vi "Main.vi"(9 "Robot Initial Position\nFrom Simulator SW corner":T1={"East"=20.0, "North"=20.0}, 10 "Simulator Bounds":T2={"Simulator E Range"=20.0, "Simulator E Min"=-10.0, "Simulator N Range"=20.0, "Simulator N Min"=-10.0}, 11 "Which Boat Am I?\n(unnecessary to set on RIO)":T3=enum."Simulation") -> ()   [LabVIEW 2011]
doc: "The main VI for Sense, Think and Act that controls the sailbot. Also includes logging code and code for communication with the OCU.\nby Olin Sailbot\noriginally by Jason Curtis"
uses:
  2-Think/2 Typedefs/Which Boat.ctl
  1,3 B-Simulation/1,3 B Typedefs/simulator bounds.ctl
  2-Think/2 Typedefs/robot velocity.ctl
  2-Think/2 Typedefs/setpoints to boat.ctl
  2-Think/2 Typedefs/sail setpt.ctl
  2-Think/2 Typedefs/rudder angle.ctl
  2-Think/2 Typedefs/UTM Circle.ctl
  0x2-OCU-Think Comm/0x2 Typedefs/Waypoints List.ctl
  2-Think/2 Classes/Waypoint/Waypoint.lvclass
  0x2-OCU-Think Comm/0x2 Typedefs/Current Waypoint.ctl
  2-Think/2 Typedefs/eStopCommand.ctl
  0x2-OCU-Think Comm/0x2 Typedefs/ocuMessage.ctl
  0x2-OCU-Think Comm/0x2 Typedefs/ocuCommands.ctl
  <vilib>/Platform/TimedLoop/XDataNode/timing_clust.ctl
  <vilib>/Platform/TimedLoop/XDataNode/nitl_modes.ctl
  <vilib>/Platform/TimedLoop/XDataNode/wakeup.ctl
  2-Think/2 Globals/2 Global.vi
  2-Think/2 Globals/2 Message Logger.vi
  <vilib>/Platform/TimedLoop/XDataNode/XDataNode.xnode
  <vilib>/Platform/TimedLoop/XDataNode/XDNodeRunTimeDep.lvlib
  0x2-OCU-Think Comm/0x2 Classes/NetworkStreams/Writer/NetworkStreamWriter.lvclass
  0x2-OCU-Think Comm/0x2 Classes/NetworkStreams/Reader/NetworkStreamReader.lvclass
  2-Think/2 Classes/Logger/Logger.lvclass
panel:
  in  "Skip Sense (->manual input only!)":bool
  in  "Enable logging?":bool=TRUE
  in  "Data storage folder":path
  out "E-stop freq.":dbl
  out "Act freq.":dbl
  out "Sense freq.":dbl
  out "Think freq.":dbl
  in  "E-Stop":bool
  # "this is the parent VI under which \nSense Think and Act run."
  # "Will save to U:\\Logs when run on the RIO"
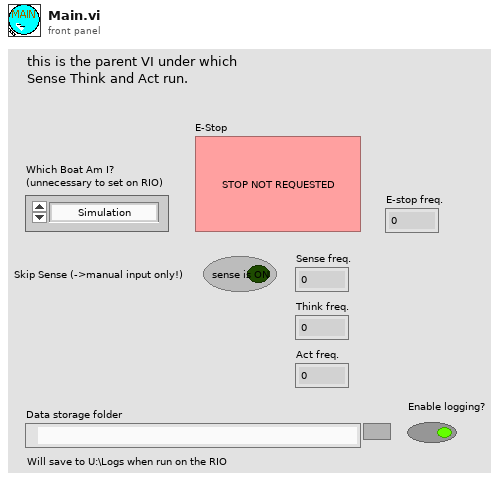
[diagram p1: front panel]
types:
  T1 = typedef "robot velocity.ctl" = cluster{"East":dbl, "North":dbl}
  T2 = typedef "simulator bounds.ctl" = cluster{"Simulator E Range":dbl, "Simulator E Min":dbl, "Simulator N Range":dbl, "Simulator N Min":dbl}
  T3 = typedef "Which Boat.ctl" = enum16{"Competition Boat", "Small RC", "Simulation"}
  T4 = typedef "setpoints to boat.ctl" = cluster{"Sail Position":T5, "Rudder Angle":T6}
  T5 = typedef "sail setpt.ctl" = dbl
  T6 = typedef "rudder angle.ctl" = dbl
  T7 = typedef "UTM Circle.ctl" = cluster{"UTM Zone":dbl, "Hemisphere":enum16{"North", "South"}, "East":dbl, "North":dbl, "Radius":dbl}
  T8 = typedef "Waypoints List.ctl" = refnum<class "Waypoint.lvclass">[]
  T9 = typedef "Current Waypoint.ctl" = i32
  T10 = typedef "eStopCommand.ctl" = enum16{"Reset E-Stop", "Get E-Stop", "Set E-Stop"}
  T11 = typedef "ocuMessage.ctl" = cluster{"OCU Command":T12, "Data":variant}
  T12 = typedef "ocuCommands.ctl" = enum16{"Pass", "Send override", "Add waypoint", "Set waypoint number", "Stop", "Add Mission", "Reset Missions/Waypts", "Edit Control Values", "Add Global No-Sail", "Log Message"}
  T13 = typedef "XDNodeRunTimeDep.lvlib/timing_clust.ctl" = cluster{"Expected End [f-1]":u64, "Actual End [f-1]":u64, "Finished Late? [f-1]":bool, "Expected End [i-1]":u64, "Actual End [i-1]":u64, "Finished Late? [i-1]":bool, "Expected Start [i]":u64, "Actual Start [i]":u64, "Expected Start [f]":u64, "Actual Start [f]":u64, "Source Name":string, "Structure Name":string, "Period":i64, "Deadline":i64, "Offset":i64, "Start":i64, "Priority":i32, "Timeout":i32, "Mode":T14, "Wakeup Reason":T15, "Error":errorcluster, "Source Type":string, "Secondary Source Type":string, "Global End Time":u64, "Global Start Time":u64, "Frame Duration":u64, "Iteration Duration":u64, "Assigned CPU":i32, "I/O Scan Engine Mode":u32}
  T14 = typedef "XDNodeRunTimeDep.lvlib/nitl_modes.ctl" = enum32{"No Change", "Process missed periods, maintain original phase", "Discard missed periods, maintain original phase", "Process missed periods, ignore original phase", "Discard missed periods, ignore original phase"}
  T15 = typedef "XDNodeRunTimeDep.lvlib/wakeup.ctl" = enum32{"Normal", "Aborted", "Asynchronous wakeup", "Timing source error", "Timed loop error", "Timeout"}
  T16 = typedef "IMAQ Image.ctl" = refnum<image>
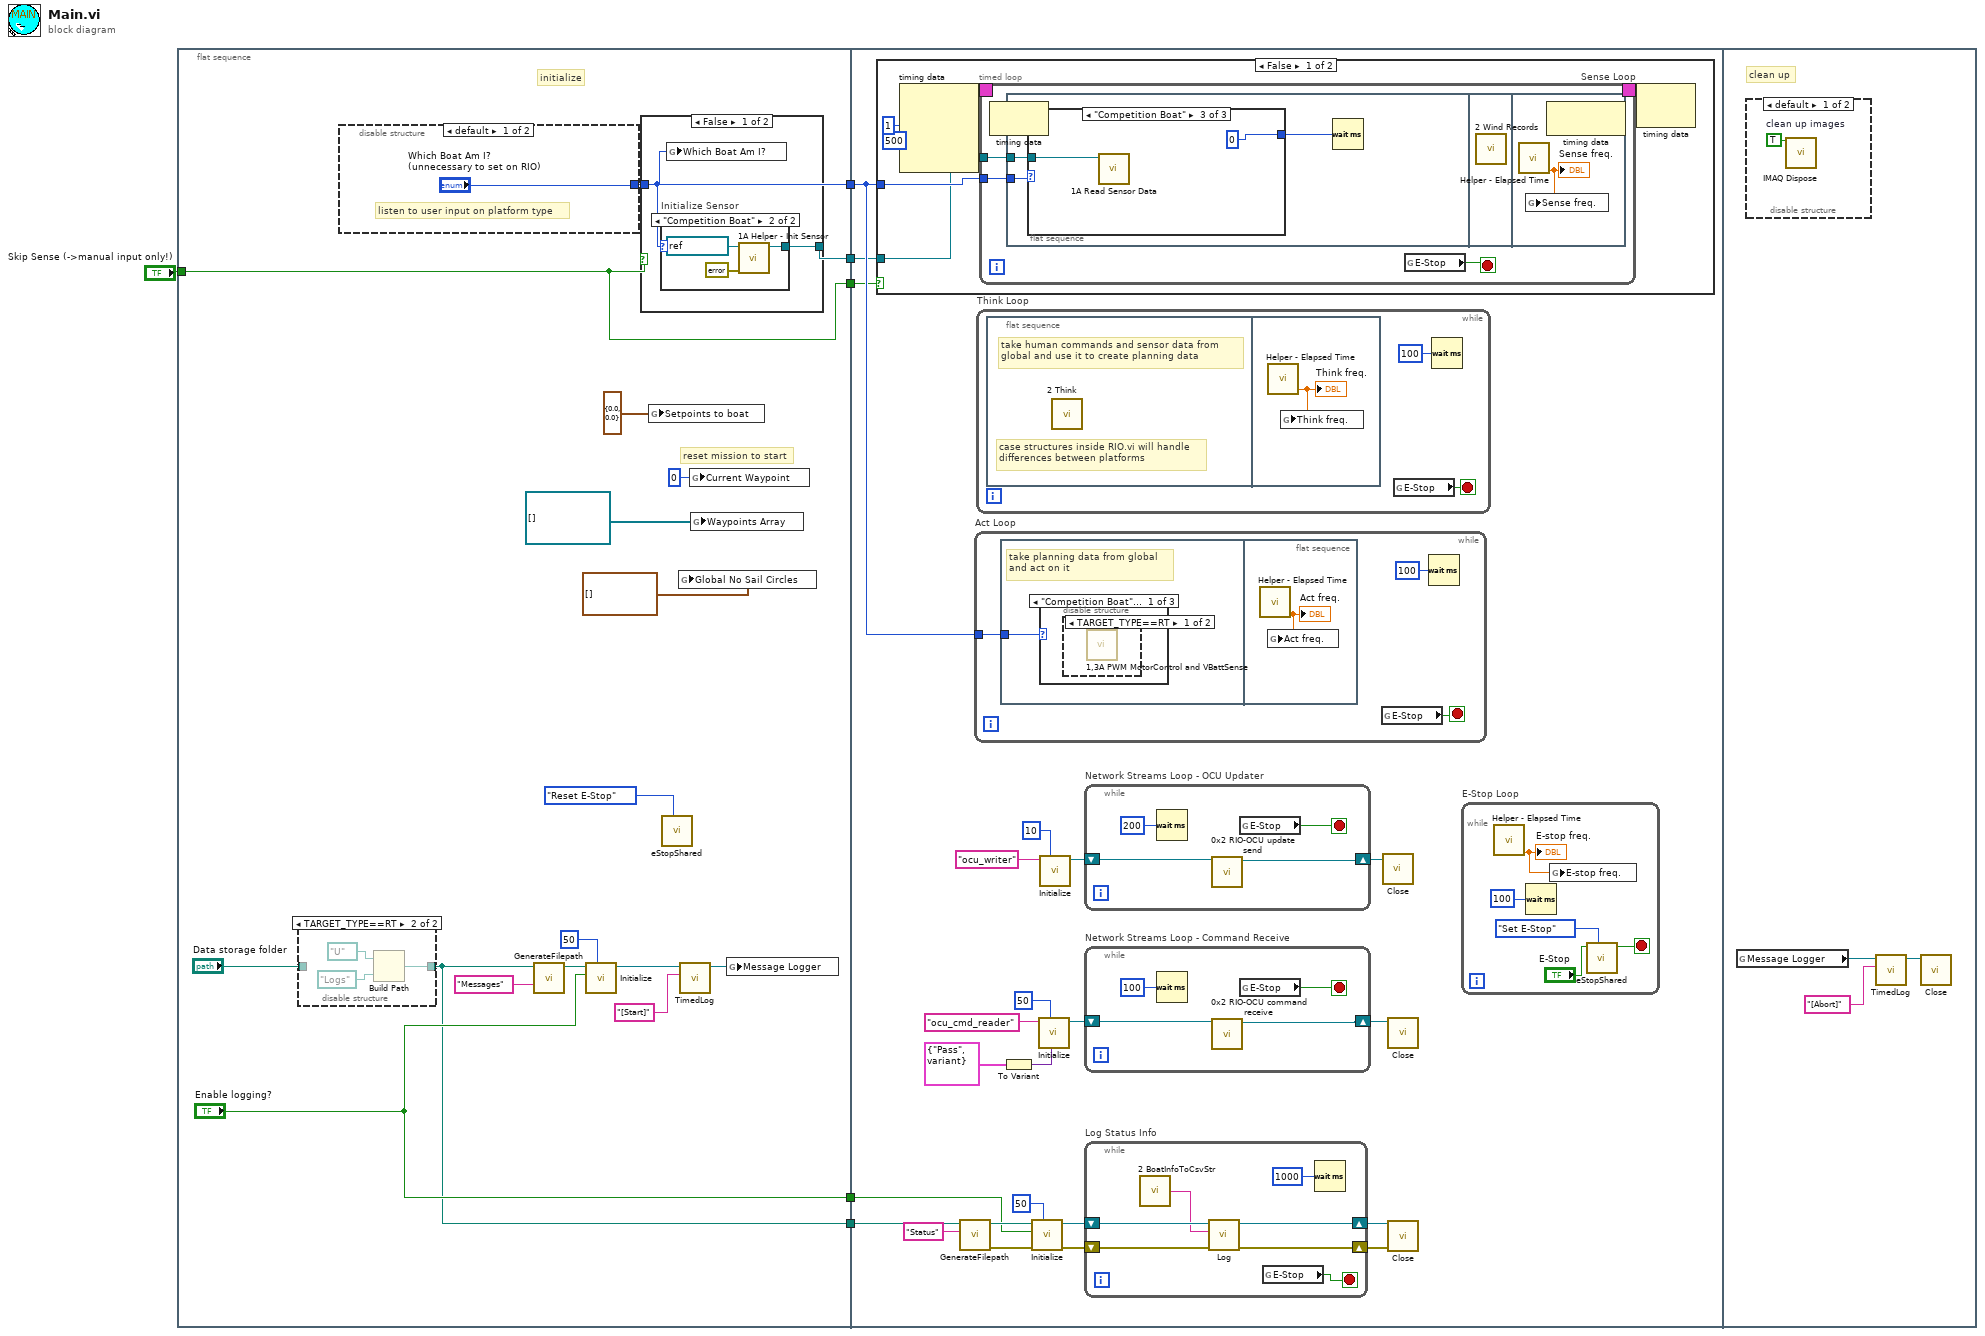
[diagram p0: block diagram]
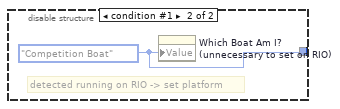
[diagram p5: hidden frame]
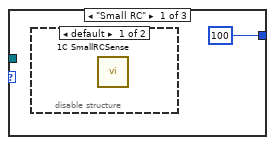
[diagram p6: hidden frame]
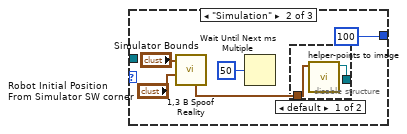
[diagram p8: hidden frame]
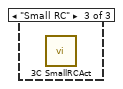
[diagram p13: hidden frame]
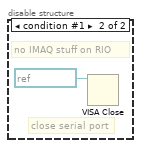
[diagram p14: hidden frame]
diagram:
  n1 = flat-sequence {
    tunnel: [w20] -> w6
    tunnel: [w21] -> w5
    tunnel: [w14] -> w4
    tunnel: ["Enable logging?"] -> w3
    tunnel: "Skip Sense (->manual input only!)" -> [w12]
    tunnel: [w12] -> w1
    tunnel: w6 -> [w57]
    tunnel: w5 -> [w56]
    tunnel: w4 -> [w40]
    tunnel: w3 -> [w36]
    tunnel: w1 -> [w35]
    frame #0 {
      # "reset mission to start"
      # "initialize"
      n2 = disable-structure shown="TARGET_TYPE==RT" {
        disable-tunnel: "Data storage folder" -> [w29 _]
        disable-tunnel: [w29 w30] -> w14
        frame condition #0 (active) {
        }
        frame condition #1 {
          n3 = Build Path(base path=path "U:/" ("Data storage folder"), name or relative path=path "Logs" ("Data storage folder")) -> (appended path=w30:path)
        }
      }
      n4 = disable-structure shown="default" {
        disable-tunnel: ["Which Boat Am I?\n(unnecessary to set on RIO)" w34] -> w20
        frame condition #0 (active) {
          # "listen to user input on platform type"
        }
        frame condition #1 {
          w34 = Which_Boat."Competition Boat" ("Which Boat Am I?")
          # "detected running on RIO -> set platform"
          n5 = property on="Which Boat Am I?\n(unnecessary to set on RIO)" class="Enum (strict)"("Value"=w34) -> ()  [unwired: 2 in, 2 out]
        }
      }
      n6 = call "GenerateFilepath.vi"("Identifier"="Messages", "Data storage folder"=w14) -> ("File path out"=w17:path)  [unwired: 8 in, 1 out]
      n7 = call "Initialize.vi"("buffer size"=50, "Enable? (T)"="Enable logging?", "File path"=w17) -> ("Logger out"=w9:refnum<class "Logger.lvclass">)  [unwired: 7 in, 1 out]
      n8 = case shown="False" w12 {
        tunnel: [w25 _] -> w21
        tunnel: w20 -> [w24 _]
        frame False {
          n9 = case "Initialize Sensor" shown="\"Competition Boat\"" w24 {
            tunnel: [_ w26] -> w25
            frame Default {
            }
            frame "Competition Boat" {
              n10 = call "1A Helper - Init Sensor.vi"("error in (no error)"=errorcluster {"status"=FALSE, "code"=0, "source"=""}, "VISA Refnum in"=refnum<visa-resource-name> "COM1" ("VISA resource name")) -> ("VISA Refnum out"=w26:refnum<visa-resource-name>)  [unwired: 7 in, 2 out]
            }
          }
          n11 = global write "2 Global.vi" "Which Boat Am I?"(w24) -> ()
        }
        frame True {
        }
      }
      n12 = global write "2 Global.vi" "Setpoints to boat"(T4 {"Sail Position"=0.0, "Rudder Angle"=0.0} ("Setpoints to boat")) -> ()
      n13 = call "eStopShared.vi"("Command"=eStopCommand."Reset E-Stop") -> ()  [unwired: 9 in, 2 out]
      n14 = global write "2 Global.vi" "Global No Sail Circles"(T7[] [] ("Global No Sail Circles")) -> ()
      n15 = call "TimedLog.vi"("Message"="[Start]", "Logger in"=w9) -> ("Logger out"=w8:refnum<class "Logger.lvclass">)  [unwired: 7 in, 2 out]
      n16 = global write "2 Global.vi" "Current Waypoint"(T9 0 ("Current Waypoint")) -> ()
      n17 = global write "2 Global.vi" "Waypoints Array"(T8 [] ("Waypoints Array")) -> ()
      n18 = global write "2 Message Logger.vi" "Message Logger"(w8) -> ()
    }
    frame #1 {
      n19 = case shown="False" w35 {
        tunnel: w57 -> [w61 _]
        tunnel: w56 -> [w60 _]
        frame False {
          n20 = node-c288(i64 1 ("Period"), 500 ("Priority")) -> (w63:T13)  [unwired: 2 in]
          n21 = timed-loop "Sense Loop" {
            tunnel: w61 -> [w65]
            tunnel: w60 -> [w64]
            timing: w63 -> [_]
            timing-out: [_] -> w62
            stop <- w66 stop-if-true
            n22 = node-c288() -> ()  [unwired: 1 in, 1 out]
            n23 = flat-sequence {
              tunnel: w65 -> [w71]
              tunnel: w64 -> [w69]
              frame #0 {
                n24 = case shown="\"Competition Boat\"" w71 {
                  tunnel: [u32 100 ("millisecond multiple") u32 100 ("millisecond multiple") u32 0 ("millisecond multiple")] -> w70
                  tunnel: w69 -> [_ _ w80]
                  frame "Small RC" {
                    n25 = disable-structure shown="default" {
                      frame condition #0 (active) {
                        n26 = call "1C SmallRCSense.vi"() -> ()  [unwired: 6 in, 6 out]
                      }
                      frame condition #1 {
                      }
                    }
                  }
                  frame "Simulation" {
                    n27 = call "1,3 B Spoof Reality.vi"("Robot Initial Position\nFrom Simulator SW corner"="Robot Initial Position\nFrom Simulator SW corner", "Simulator Bounds"="Simulator Bounds") -> ("Boat Path"=w76:cluster{"X Position":dbl, "Y Position":dbl}[])  [unwired: 3 in, 6 out]
                    n28 = Wait Until Next ms Multiple(millisecond multiple=u32 50) -> ()  [unwired: 1 out]
                    n29 = disable-structure shown="default" {
                      disable-tunnel: w76 -> [w79 _]
                      disable-tunnel: [w78 _] -> _
                      frame condition #0 (active) {
                        n30 = call "helper-points to image.vi"("Array of Points"=w79) -> ("Image Out"=w78:T16)  [unwired: 10 in]
                      }
                      frame condition #1 {
                        # "no IMAQ\non RIO"
                      }
                    }
                  }
                  frame "Competition Boat" {
                    n31 = call "1A Read Sensor Data.vi"("VISA resource name (in)"=w80) -> ()  [unwired: 9 in, 2 out]
                  }
                }
                n32 = Wait (ms)(milliseconds to wait=w70) -> ()  [unwired: 1 out]
              }
              frame #1 {
                n33 = call "2 Wind Records.vi"() -> ()  [unwired: 12 in]
              }
              frame #2 {
                n34 = call "Helper - Elapsed Time.vi"() -> ("Frequency (Hz)"=w82:dbl)  [unwired: 10 in, 1 out]
                "Sense freq." <- w82
                n35 = global write "2 Global.vi" "Sense freq."(w82) -> ()
              }
            }
            n36 = global read "2 Global.vi" "E-Stop"() -> (w66:bool)
            n37 = node-c288() -> ()  [unwired: 1 in, 1 out]
          }
          n38 = node-c288(w62) -> ()  [unwired: 1 out]
        }
        frame True {
          # "Sense is cancelled"
        }
      }
      n39 = call "GenerateFilepath.vi"("Identifier"="Status", "Data storage folder"=w40) -> ("error out"=w44:errorcluster, "File path out"=w45:path)  [unwired: 8 in]
      n40 = while "Act Loop" {
        tunnel: w57 -> [w112]
        stop <- w113 stop-if-true
        n41 = flat-sequence {
          tunnel: w112 -> [w114]
          frame #0 {
            # "take planning data from global\nand act on it"
            n42 = case shown="\"Competition Boat\", Default" w114 {
              frame "Competition Boat", Default {
                n43 = disable-structure shown="TARGET_TYPE==RT" {
                  frame condition #0 {
                    n44 = call "1,3A PWM MotorControl and VBattSense.vi"() -> ()  [unwired: 12 in]
                  }
                  frame condition #1 (active) {
                  }
                }
              }
              frame "Simulation" {
                # "simulation Act\nis integrated with\nsimulation Think"
              }
              frame "Small RC" {
                n45 = call "3C SmallRCAct.vi"() -> ()  [unwired: 12 in]
              }
            }
          }
          frame #1 {
            n46 = call "Helper - Elapsed Time.vi"() -> ("Frequency (Hz)"=w115:dbl)  [unwired: 10 in, 1 out]
            "Act freq." <- w115
            n47 = global write "2 Global.vi" "Act freq."(w115) -> ()
          }
        }
        n48 = global read "2 Global.vi" "E-Stop"() -> (w113:bool)
        n49 = Wait (ms)(milliseconds to wait=u32 100 ("millisecond multiple")) -> ()  [unwired: 1 out]
      }
      n50 = while "Think Loop" {
        stop <- w109 stop-if-true
        n51 = flat-sequence {
          frame #0 {
            # "case structures inside RIO.vi will handle\ndifferences between platforms"
            # "take human commands and sensor data from\nglobal and use it to create planning data"
            n52 = call "2 Think.vi"() -> ()  [unwired: 12 in]
          }
          frame #1 {
            n53 = call "Helper - Elapsed Time.vi"() -> ("Frequency (Hz)"=w110:dbl)  [unwired: 10 in, 1 out]
            "Think freq." <- w110
            n54 = global write "2 Global.vi" "Think freq."(w110) -> ()
          }
        }
        n55 = global read "2 Global.vi" "E-Stop"() -> (w109:bool)
        n56 = Wait (ms)(milliseconds to wait=u32 100 ("millisecond multiple")) -> ()  [unwired: 1 out]
      }
      n57 = To Variant(anything=T11 {"OCU Command"=enum."Pass", "Data"=variant} ("OCU Message")) -> (Variant=w51:variant)
      n58 = call "Initialize.vi"("buffer size"=50, "error in (no error)"=w44, "Enable? (T)"=w36, "File path"=w45) -> ("error out"=w41:errorcluster, "Logger out"=w42:refnum<class "Logger.lvclass">)  [unwired: 6 in]
      n59 = call "Initialize.vi"("Default return"=w51, "reader buffer size"=50 ("writer buffer size"), "reader name"="ocu_cmd_reader") -> ("NetworkStreamWriter out"=w47:refnum<class "NetworkStreamReader.lvclass">)  [unwired: 6 in, 2 out]
      n60 = call "Initialize.vi"("writer buffer size"=10, "writer name"="ocu_writer") -> ("NetworkStreamWriter out"=w55:refnum<class "NetworkStreamWriter.lvclass">)  [unwired: 7 in, 2 out]
      n61 = while "Network Streams Loop - OCU Updater" {
        shift-right: [w99] -> w54
        shift-left: w55 -> [w100]
        stop <- w102 stop-if-true
        n62 = Wait (ms)(milliseconds to wait=u32 200 ("millisecond multiple")) -> ()  [unwired: 1 out]
        n63 = call "0x2 RIO-OCU update send.vi"("OCU Writer In"=w100) -> ("OCU Writer Out"=w99:refnum<class "NetworkStreamWriter.lvclass">)  [unwired: 10 in]
        n64 = global read "2 Global.vi" "E-Stop"() -> (w102:bool)
      }
      n65 = while "Network Streams Loop - Command Receive" {
        shift-right: [w95] -> w48
        shift-left: w47 -> [w96]
        stop <- w98 stop-if-true
        n66 = Wait (ms)(milliseconds to wait=u32 100 ("millisecond multiple")) -> ()  [unwired: 1 out]
        n67 = call "0x2 RIO-OCU command receive.vi"("Manual Override Reader In"=w96) -> ("Manual Override Reader Out"=w95:refnum<class "NetworkStreamReader.lvclass">)  [unwired: 10 in]
        n68 = global read "2 Global.vi" "E-Stop"() -> (w98:bool)
      }
      n69 = while "Log Status Info" {
        shift-right: [w92] -> w38
        shift-left: w42 -> [w93]
        shift-right: [w91] -> w37
        shift-left: w41 -> [w90]
        stop <- w94 stop-if-true
        n70 = call "2 BoatInfoToCsvStr.vi"() -> ("Log String"=w88:string)  [unwired: 1 in]
        n71 = call "Log.vi"("error in (no error)"=w90, "Message"=w88, "Logger in"=w93) -> ("error out"=w91:errorcluster, "Logger out"=w92:refnum<class "Logger.lvclass">)  [unwired: 7 in]
        n72 = global read "2 Global.vi" "E-Stop"() -> (w94:bool)
        n73 = Wait (ms)(milliseconds to wait=u32 1000 ("millisecond multiple")) -> ()  [unwired: 1 out]
      }
      n74 = call "Close.vi"("NetworkStreamWriter in"=w54) -> ()  [unwired: 9 in, 2 out]
      n75 = call "Close.vi"("NetworkStreamReader in"=w48) -> ()  [unwired: 9 in, 2 out]
      n76 = call "Close.vi"("error in (no error)"=w37, "NetworkStreamWriter in"=w38) -> ()  [unwired: 9 in, 1 out]
      n77 = while "E-Stop Loop" {
        stop <- w104 stop-if-true
        n78 = call "Helper - Elapsed Time.vi"() -> ("Frequency (Hz)"=w103:dbl)  [unwired: 10 in, 1 out]
        "E-stop freq." <- w103
        n79 = Wait (ms)(milliseconds to wait=u32 100 ("millisecond multiple")) -> ()  [unwired: 1 out]
        n80 = global write "2 Global.vi" "E-stop freq."(w103) -> ()
        n81 = call "eStopShared.vi"("Command"=eStopCommand."Set E-Stop", "E-Stop"="E-Stop") -> ("E-Stop Out"=w104:bool)  [unwired: 8 in, 1 out]
      }
    }
    frame #2 {
      # "clean up"
      n82 = global read "2 Message Logger.vi" "Message Logger"() -> (w118:refnum<class "Logger.lvclass">)
      n83 = disable-structure shown="default" {
        frame condition #0 (active) {
          w119 = TRUE  # clean up images
          n84 = call "IMAQ Dispose"("All Images? (No)"=w119) -> ()  [unwired: 5 in, 1 out]
        }
        frame condition #1 {
          # "close serial port"
          # "no IMAQ stuff on RIO"
          n85 = VISA Close(VISA resource name=refnum<visa-resource-name> "COM1") -> ()  [unwired: 1 in, 1 out]
        }
      }
      n86 = call "TimedLog.vi"("Message"="[Abort]", "Logger in"=w118) -> ("Logger out"=w116:refnum<class "Logger.lvclass">)  [unwired: 7 in, 2 out]
      n87 = call "Close.vi"("NetworkStreamWriter in"=w116) -> ()  [unwired: 10 in, 1 out]
    }
  }
